vi "Add Test to Recent Tests.vi"(9 "New Test":string, 10 "Recent Tests":string) -> (2 "Recent Tests":string)   [LabVIEW 2009]
uses:
  <userlib>/_OpenG.lib/array/array.llb/Remove Duplicates from 1D Array (String)__ogtk.vi
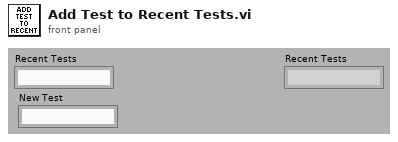
[diagram p1: front panel]
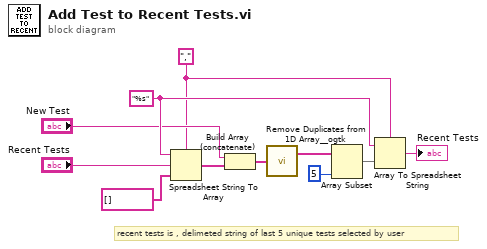
[diagram p0: block diagram]
diagram:
  w1 = "," ("delimiter (Tab)")
  w8 = "%s" ("format string")
  # "recent tests is , delimeted string of last 5 unique tests selected by user"
  n1 = Spreadsheet String To Array(delimiter (Tab)=w1, format string=w8, spreadsheet string="Recent Tests", array type (2D Dbl)=string[] []) -> (array=w6:string[])
  n2 = Build Array (concatenate)("New Test", w6) -> (w3:string[])
  n3 = call-poly <userlib>:"Remove Duplicates from 1D Array__ogtk.vi"("Input Array"=w3) -> ("Output Array"=w2:string[])  [unwired: 1 out]
  n4 = Array Subset(array=w2, length=5) -> (w11:string[])  [unwired: 1 in]
  n5 = Array To Spreadsheet String(delimiter (Tab)=w1, array=w11, 3:w8) -> (spreadsheet string=→"Recent Tests":string)
